vi "target.vi"() -> ()   [LabVIEW 2020]
uses:
  <vilib>/Platform/TimedLoop/XDataNode/timing_clust.ctl
  <vilib>/Platform/TimedLoop/XDataNode/nitl_modes.ctl
  <vilib>/Platform/TimedLoop/XDataNode/wakeup.ctl
  <vilib>/rvi/Emulation/niFpgaSctlEmulationGetInTimedLoop.vi
  <vilib>/rvi/Emulation/niFpgaEmulationReportErrorSimple.vi
  <vilib>/rvi/Emulation/niFpgaGetClockAttributes.vi
  <vilib>/rvi/Emulation/niFpgaCriticalErrorInLSC.vi
  <vilib>/rvi/interface/RandomDataEmulation/niFpgaRandomDataHandleErrors.vi
  <vilib>/Platform/TimedLoop/XDataNode/XDataNode.xnode
  <vilib>/rvi/DataTransferAndStorage/Container/XNode/niFpgaContainer.xnode
  <vilib>/rvi/interface/RandomDataEmulation/nirviRandomDataFpgaReadWriteTemplate.vi
  <vilib>/Platform/TimedLoop/XDataNode/XDNodeRunTimeDep.lvlib
panel:
  out "Timed Out? FIFO out index":bool
  out "Timed Out? FIFO out IMG":bool
  out "Timed Out? FIFO out REAL":bool
  out "Timed Out? FIFO in REAL":bool
  out "Timed Out? FIFO in IMG":bool
  out "sort time (us)":u32
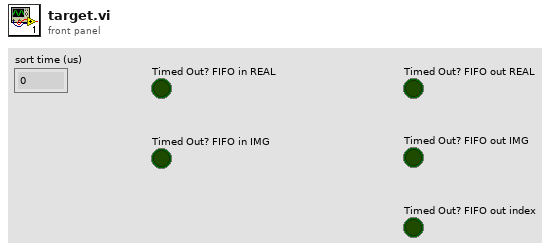
[diagram p1: front panel]
types:
  T1 = typedef "XDNodeRunTimeDep.lvlib/timing_clust.ctl" = cluster{"Expected End [f-1]":u64, "Actual End [f-1]":u64, "Finished Late? [f-1]":bool, "Expected End [i-1]":u64, "Actual End [i-1]":u64, "Finished Late? [i-1]":bool, "Expected Start [i]":u64, "Actual Start [i]":u64, "Expected Start [f]":u64, "Actual Start [f]":u64, "Source Name":string, "Structure Name":string, "Period":i64, "Deadline":i64, "Offset":i64, "Start":i64, "Priority":i32, "Timeout":i32, "Mode":T2, "Wakeup Reason":T3, "Error":errorcluster, "Source Type":string, "Secondary Source Type":string, "Global End Time":u64, "Global Start Time":u64, "Frame Duration":u64, "Iteration Duration":u64, "Assigned CPU":i32, "I/O Scan Engine Mode":u32}
  T2 = typedef "XDNodeRunTimeDep.lvlib/nitl_modes.ctl" = enum32{"No Change", "Process missed periods, maintain original phase", "Discard missed periods, maintain original phase", "Process missed periods, ignore original phase", "Discard missed periods, ignore original phase"}
  T3 = typedef "XDNodeRunTimeDep.lvlib/wakeup.ctl" = enum32{"Normal", "Aborted", "Asynchronous wakeup", "Timing source error", "Timed loop error", "Timeout"}
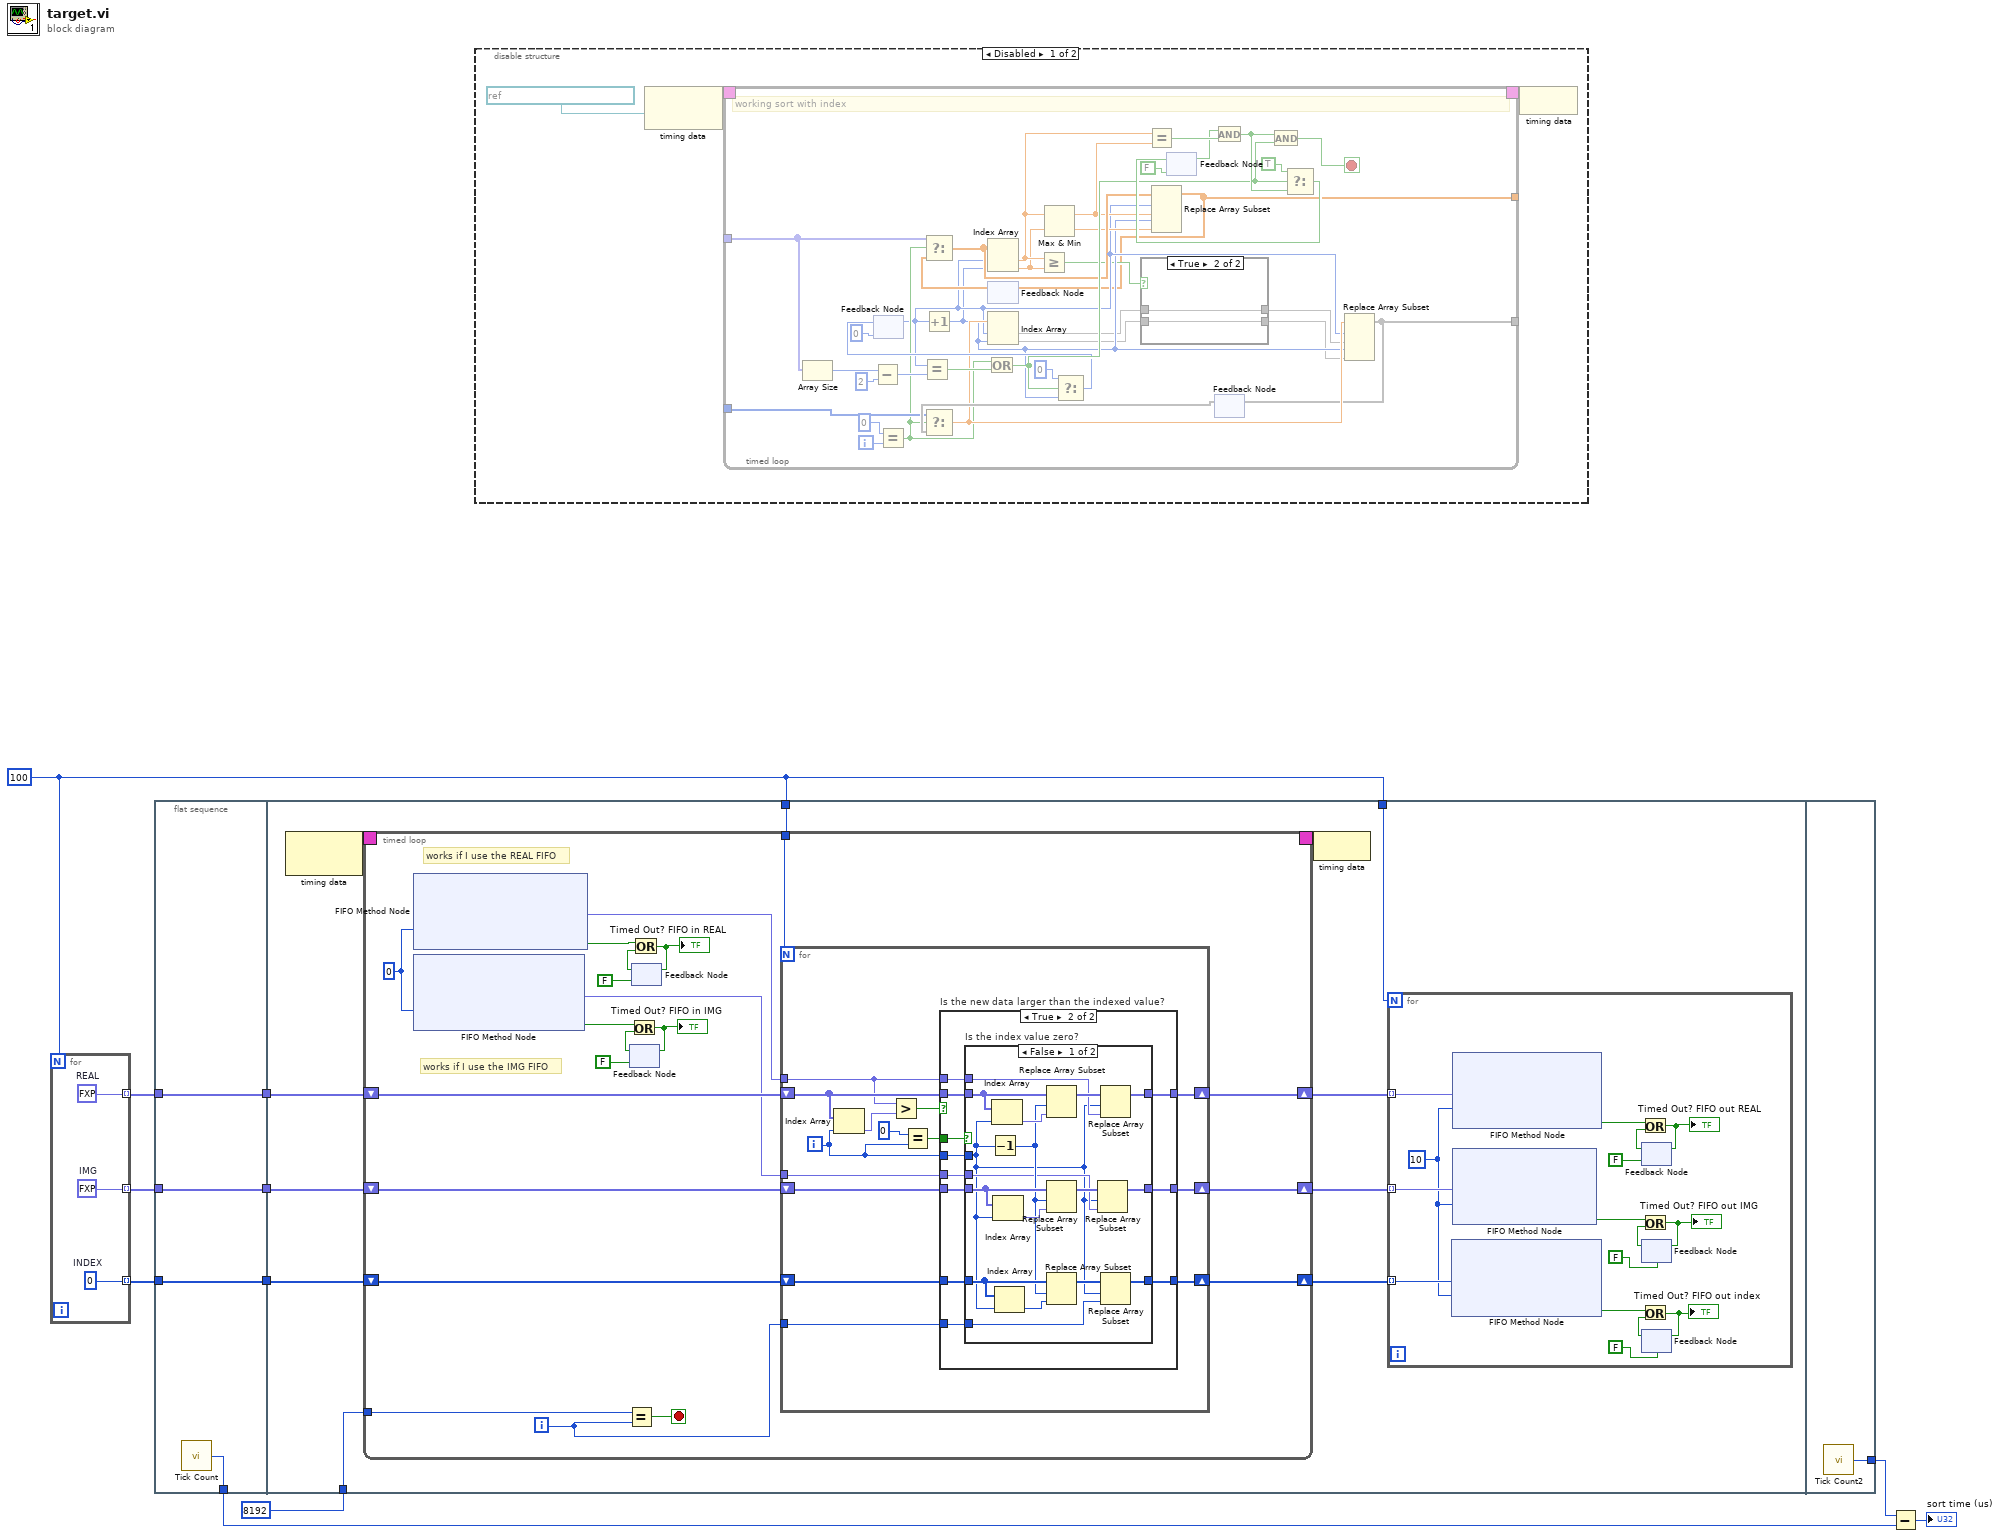
[diagram p0: block diagram]
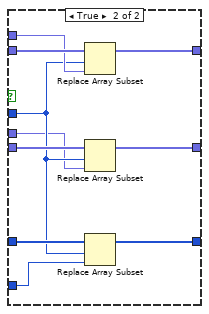
[diagram p5: hidden frame]
diagram:
  w3 = 100
  n1 = for {
    N: w3 -> [_]
    tunnel: [w14] -> w5 mode=indexing
    tunnel: [w13] -> w7 mode=indexing
    tunnel: [w12] -> w1 mode=indexing
    w12 = fxp<+/-,32,21> 0.0  # IMG
    w13 = 0  # INDEX
    w14 = fxp<+/-,32,21> 0.0  # REAL
  }
  n2 = flat-sequence {
    tunnel: [w18] -> w10
    tunnel: [w17] -> w8
    tunnel: w7 -> [w17]
    tunnel: [w16] -> w6
    tunnel: w5 -> [w16]
    tunnel: [w15] -> w2
    tunnel: w1 -> [w15]
    tunnel: w8 -> [w29]
    tunnel: w6 -> [w28]
    tunnel: 8192 ("samples") -> [w26]
    tunnel: w3 -> [w27]
    tunnel: w3 -> [w23]
    tunnel: w2 -> [w19]
    tunnel: [w126] -> w11
    frame #0 {
      n3 = call "Tick Count"() -> ("Tick Count(uSec)"=w18:u32)
    }
    frame #1 {
      n4 = node-c288() -> (w25:T1)  [unwired: 1 in]
      n5 = timed-loop {
        shift-right: [w65] -> w21
        shift-left: w28 -> [w66]
        shift-right: [w64] -> w22
        shift-left: w29 -> [w63]
        tunnel: w27 -> [w62]
        tunnel: w26 -> [w60]
        timing: w25 -> [_]
        timing-out: [_] -> w24
        shift-right: [w58] -> w20
        shift-left: w19 -> [w57]
        i -> [w61]
        stop <- w59 stop-if-true
        w56 = 0 ("Timeout")
        # "works if I use the REAL FIFO"
        # "works if I use the IMG FIFO"
        n6 = xnode ("FIFO Method Node")("Timeout"=w56) -> ("Element"=w54:fxp<+/-,32,21>, "Timed Out?"=w46:bool)  [unwired: 1 in, 1 out]
        n7 = xnode ("FIFO Method Node")("Timeout"=w56) -> ("Element"=w55:fxp<+/-,32,21>, "Timed Out?"=w50:bool)  [unwired: 1 in, 1 out]
        n8 = Equal?(x=w60, y=w61) -> (x = y?=w59:bool)
        n9 = feedback #1(FALSE) -> (w51:bool)
        n10 = Or(x=w50, y=w51) -> (x .or. y?=w52:bool)
        "Timed Out? FIFO in IMG" <- w52
        n11 = feedback-in #1(w52) -> ()
        n12 = feedback #2(FALSE) -> (w47:bool)
        n13 = Or(x=w46, y=w47) -> (x .or. y?=w48:bool)
        "Timed Out? FIFO in REAL" <- w48
        n14 = feedback-in #2(w48) -> ()
        n15 = for {
          N: w62 -> [_]
          tunnel: w54 -> [w77]
          shift-right: [w76] -> w65
          shift-left: w66 -> [w78]
          tunnel: w61 -> [w74]
          shift-right: [w72] -> w64
          shift-left: w63 -> [w73]
          shift-right: [w69] -> w58
          shift-left: w57 -> [w68]
          tunnel: w55 -> [w67]
          i -> [w75]
          n16 = Index Array(array=w78, index=w75) -> (element=w80:fxp<+/-,32,21>)
          n17 = Greater?(x=w77, y=w80) -> (0:w79:bool)
          n18 = Equal?(x=0, y=w75) -> (x = y?=w70:bool)
          n19 = case "Is the new data larger than the indexed value?" shown="True" w79 {
            tunnel: w78 -> [w83 w93]
            tunnel: w70 -> [_ w94]
            tunnel: w77 -> [_ w92]
            tunnel: w75 -> [_ w91]
            tunnel: [w83 w90] -> w76
            tunnel: w74 -> [_ w89]
            tunnel: w73 -> [w82 w88]
            tunnel: [w82 w87] -> w72
            tunnel: [w81 w86] -> w69
            tunnel: w68 -> [w81 w85]
            tunnel: w67 -> [_ w84]
            frame False {
            }
            frame True {
              n20 = case "Is the index value zero?" shown="False" w94 {
                tunnel: w93 -> [w111 w121]
                tunnel: w92 -> [w108 w120]
                tunnel: w91 -> [w95 w114]
                tunnel: [w107 w119] -> w90
                tunnel: w89 -> [w102 w118]
                tunnel: w88 -> [w104 w117]
                tunnel: [w103 w116] -> w87
                tunnel: [w97 w112] -> w86
                tunnel: w85 -> [w101 w115]
                tunnel: w84 -> [w96 w113]
                frame False {
                  n21 = Decrement(x=w95) -> (x-1=w99:i32)
                  n22 = Index Array(array=w111, index=w95) -> (element=w110:fxp<+/-,32,21>)
                  n23 = Index Array(array=w101, index=w95) -> (element=w100:fxp<+/-,32,21>)
                  n24 = Index Array(array=w104, index=w95) -> (element=w106:i32)
                  n25 = Replace Array Subset(array=w111, new element=w110, index=w99) -> (w109:fxp<+/-,32,21>[])
                  n26 = Replace Array Subset(array=w101, new element=w100, index=w99) -> (w98:fxp<+/-,32,21>[])
                  n27 = Replace Array Subset(array=w104, new element=w106, index=w99) -> (w105:i32[])
                  n28 = Replace Array Subset(array=w98, new element=w96, index=w95) -> (w97:fxp<+/-,32,21>[])
                  n29 = Replace Array Subset(array=w109, new element=w108, index=w95) -> (w107:fxp<+/-,32,21>[])
                  n30 = Replace Array Subset(array=w105, new element=w102, index=w95) -> (w103:i32[])
                }
                frame True {
                  n31 = Replace Array Subset(array=w121, new element=w120, index=w114) -> (w119:fxp<+/-,32,21>[])
                  n32 = Replace Array Subset(array=w115, new element=w113, index=w114) -> (w112:fxp<+/-,32,21>[])
                  n33 = Replace Array Subset(array=w117, new element=w118, index=w114) -> (w116:i32[])
                }
              }
            }
          }
        }
      }
      n34 = node-c288(w24) -> ()
      n35 = for {
        N: w23 -> [_]
        tunnel: w22 -> [w45] mode=indexing
        tunnel: w21 -> [w44] mode=indexing
        tunnel: w20 -> [w43] mode=indexing
        w42 = 10 ("Timeout")
        n36 = xnode ("FIFO Method Node")("Element"=w45, "Timeout"=w42) -> ("Timed Out?"=w30:bool)  [unwired: 1 in, 1 out]
        n37 = xnode ("FIFO Method Node")("Element"=w44, "Timeout"=w42) -> ("Timed Out?"=w38:bool)  [unwired: 1 in, 1 out]
        n38 = xnode ("FIFO Method Node")("Element"=w43, "Timeout"=w42) -> ("Timed Out?"=w34:bool)  [unwired: 1 in, 1 out]
        n39 = feedback #3(FALSE) -> (w39:bool)
        n40 = Or(x=w38, y=w39) -> (x .or. y?=w40:bool)
        "Timed Out? FIFO out REAL" <- w40
        n41 = feedback-in #3(w40) -> ()
        n42 = feedback #4(FALSE) -> (w37:bool)
        n43 = Or(x=w34, y=w37) -> (x .or. y?=w36:bool)
        "Timed Out? FIFO out IMG" <- w36
        n44 = feedback-in #4(w36) -> ()
        n45 = feedback #5(FALSE) -> (w33:bool)
        n46 = Or(x=w30, y=w33) -> (x .or. y?=w32:bool)
        "Timed Out? FIFO out index" <- w32
        n47 = feedback-in #5(w32) -> ()
      }
    }
    frame #2 {
      n48 = call "Tick Count2"() -> ("Tick Count(uSec)"=w126:u32)
    }
  }
  n49 = disable-structure shown="Disabled" {
    frame Disabled {
      n50 = node-c288(refnum<k21> "40 MHz Onboard Clock" ("Source Name")) -> (w130:T1)
      n51 = timed-loop {
        tunnel: _ -> [w164]
        tunnel: [w143] -> w128
        timing: w130 -> [_]
        timing-out: [_] -> w129
        tunnel: [w132] -> _
        tunnel: [w131] -> _
        i -> [w147]
        stop <- w148 stop-if-true
        # "working sort with index"
        n52 = Array Size(array=w164) -> (size(s)=w167:i32)
        n53 = Subtract(x=w167, y=2) -> (x-y=w165:i32)
        n54 = feedback #6(0 ("y")) -> (w141:i32)
        n55 = Equal?(x=0, y=w147) -> (x = y?=w142:bool)
        n56 = Equal?(x=w141, y=w165) -> (x = y?=w152:bool)
        n57 = Increment(x=w141) -> (x+1=w140:i32)
        n58 = Or(x=w142, y=w152) -> (x .or. y?=w155:bool)
        n59 = feedback #7() -> (w157:dbl[])  [unwired: 1 in]
        n60 = Select(t=w164, s=w142, f=w157) -> (s? t:f=w151:dbl[])
        n61 = Index Array(array=w151, index #1=w141, index #2=w140) -> (element #1=w135:dbl, element #2=w134:dbl)
        n62 = Greater Or Equal?(x=w135, y=w134) -> (x >= y?=w133:bool)
        n63 = Max & Min(x=w135, y=w134) -> (max(x,y)=w150:dbl, min(x,y)=w149:dbl)
        n64 = Select(t=0 ("y"), s=w155, f=w140) -> (s? t:f=w153:i32)
        n65 = feedback-in #6(w153) -> ()
        n66 = Equal?(x=w135, y=w150) -> (x = y?=w163:bool)
        n67 = Replace Array Subset(array=w151, new element #1=w150, index #1=w141, new element #2=w149, index #2=w140) -> (w132:dbl[])
        n68 = feedback-in #7(w132) -> ()
        n69 = feedback #8(FALSE ("t")) -> (w160:bool)
        n70 = And(x=w160, y=w163) -> (x .and. y?=w158:bool)
        n71 = feedback #9() -> (w145:void[])  [unwired: 1 in]
        n72 = Select(t=w143, s=w142, f=w145) -> (s? t:f=w144:dbl)
        n73 = Index Array(array=w144, index #1=w141, index #2=w140) -> (element #1=w139, element #2=w136)
        n74 = case shown="True" w133 {
          tunnel: w139 -> [w169 w171]
          tunnel: [w168 w171] -> w138
          tunnel: [w169 w170] -> w137
          tunnel: w136 -> [w168 w170]
          frame False {
          }
          frame True {
          }
        }
        n75 = And(x=w158, y=w155) -> (x .and. y?=w148:bool)
        n76 = Select(t=TRUE, s=w155, f=w158) -> (s? t:f=w161:bool)
        n77 = feedback-in #8(w161) -> ()
        n78 = Replace Array Subset(array=w144, new element #1=w138, index #1=w141, new element #2=w137, index #2=w140) -> (w131:void[])
        n79 = feedback-in #9(w131) -> ()
      }
      n80 = node-c288(w129) -> ()
    }
    frame Enabled {
    }
  }
  n81 = Subtract(x=w11, y=w10) -> (x-y=→"sort time (us)":u32)
